vi "Find Dose Range.vi"(0 "Dose Estimate [Gy]":dbl step=0.25) -> (1 "Dose Range [Gy]":u16(ring) items=["<0.5 Gy", "0.5 - 1.0 Gy", "1.0 - 2.0 Gy", "2.0 - 3.5 Gy", "3.5 - 5.5 Gy", "5.5 - 7.5 Gy", "7.5 - 10.0 Gy", "10.0 - 20.0 Gy", "20.0 - 30.0 Gy", ">30 Gy"], 2 "Dose Range [Gy]":string="<0.5 Gy")   [LabVIEW 2016]
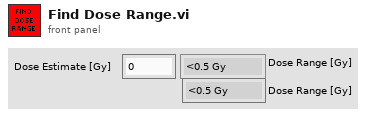
[diagram p1: front panel]
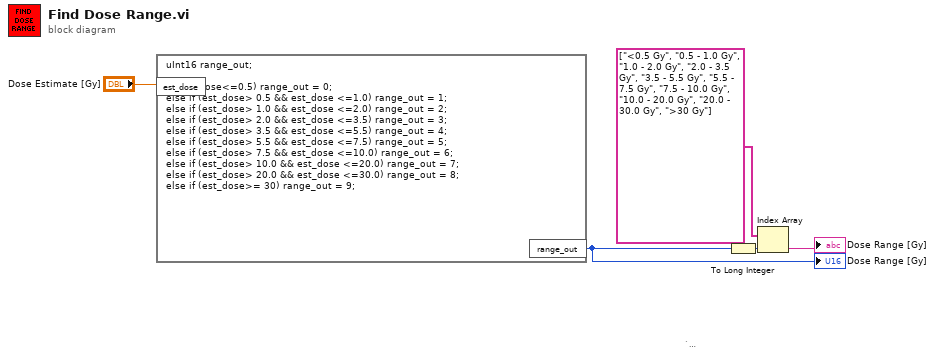
[diagram p0: block diagram]
diagram:
  # "``"
  n1 = formula code="uInt16 range_out;\n\nif (est_dose<=0.5) range_out = 0;\nelse if (est_dose> 0.5 && est_dose <=1.0) range_out = 1;\nelse if (est_dose> 1.0 && est_dose <=2.0) range_out = 2;\nelse if (est_dose> 2.0 && est_dose <=3.5) range_out = 3;\nelse if (est_dose> 3.5 && est_dose <=5.5) range_out = 4;\nelse if (est_dose> 5.5 && est_dose <=7.5) range_out = 5;\nelse if (est_dose> 7.5 && est_dose <=10.0) range_out = 6;\nelse if (est_dose> 10.0 && est_dose <=20.0) range_out = 7;\nelse if (est_dose> 20.0 && est_dose <=30.0) range_out = 8;\nelse if (est_dose>= 30) range_out = 9;"("est_dose"="Dose Estimate [Gy]") -> ("range_out"=w3:u16)
  "Dose Range [Gy]" <- w3
  n2 = To Long Integer(number=w3) -> (32bit integer=w1:i32)
  n3 = Index Array(array=string[] ["<0.5 Gy", "0.5 - 1.0 Gy", "1.0 - 2.0 Gy", "2.0 - 3.5 Gy", "3.5 - 5.5 Gy", "5.5 - 7.5 Gy", "7.5 - 10.0 Gy", "10.0 - 20.0 Gy", "20.0 - 30.0 Gy", ">30 Gy"], index=w1) -> (element=→"Dose Range [Gy]":string)
